vi "Collection.vi"(8 "error in (no error)":errorcluster) -> (0 "error out":errorcluster)   [LabVIEW 2017]
uses:
  Controls/First-After.ctl
  Controls/Data Save Loop States.ctl
panel:
  out "Saving Progress":u8(slide) scale=-1.0..4.0
  out "Exit?":bool
  out "Saving":bool
  out "Recording Save Path":path
  out "Recording":bool
  in  "Home Button":bool
  in  "Record Button":bool
  out "Mic 2":dynamicdata(graph)
  out "Mic 1":dynamicdata(graph)
  out "Sensor 6":dynamicdata(graph)
  out "Sensor 4":dynamicdata(graph)
  out "Sensor 3":dynamicdata(graph)
  out "Sensor 2":dynamicdata(graph)
  out "Sensor 5":dynamicdata(graph)
  out "Sensor 1":dynamicdata(graph)
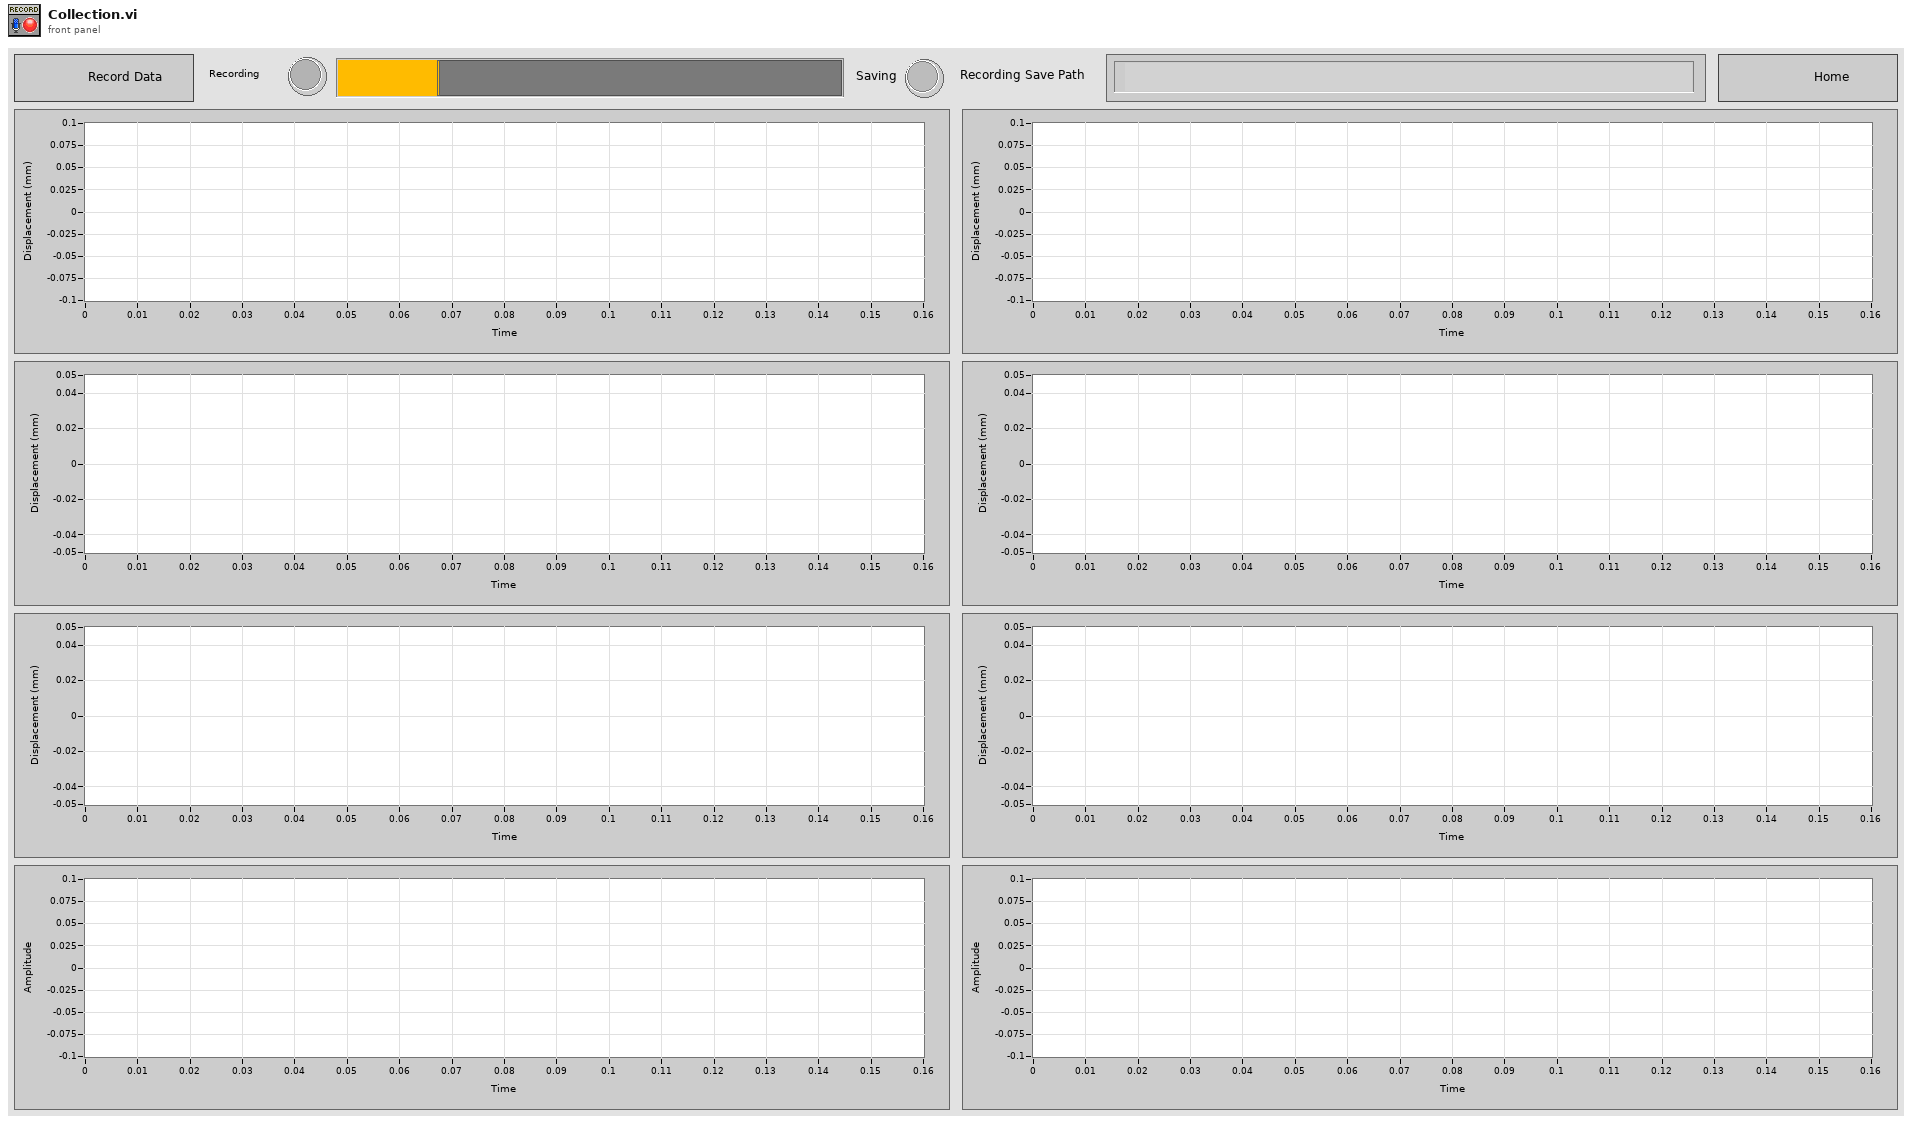
[diagram p1: front panel]
types:
  T1 = enum16{"open", "replace", "create", "open or create", "replace or create", "replace or create with confirmation"}
  T2 = typedef "Data Save Loop States.ctl" = enum16{"Waiting", "Recording", "Saving"}
  T3 = typedef "First-After.ctl" = enum16{"First", "After"}
  T4 = enum8{"Enabled", "Disabled", "Disabled and Grayed Out"}
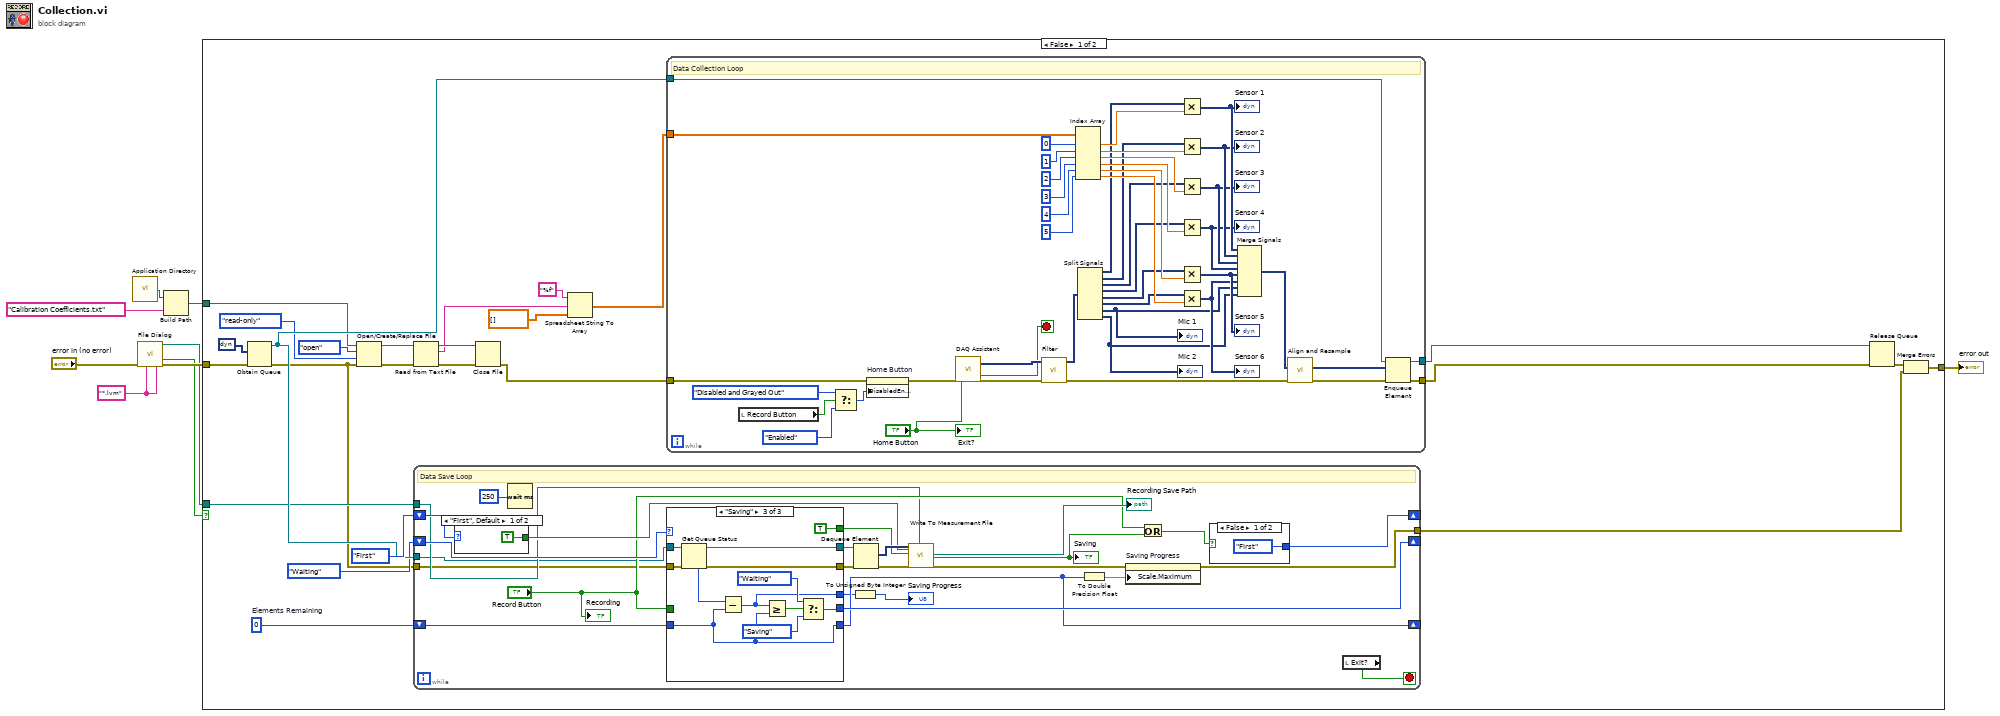
[diagram p0: block diagram]
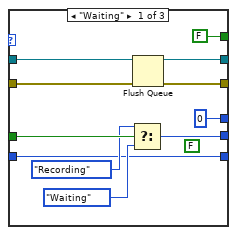
[diagram p2: hidden frame]
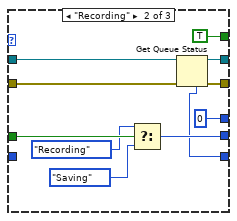
[diagram p3: hidden frame]
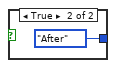
[diagram p4: hidden frame]
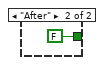
[diagram p5: hidden frame]
diagram:
  w9 = "*.lvm" ("pattern label")
  n1 = call <vilib>:"Application Directory.vi"() -> ("Application Directory"=w3:path)
  n2 = call "File Dialog"("error in"="error in (no error)", "pattern (all files)"=w9, "pattern label"=w9) -> ("selected path"=w5:path, "cancelled"=w4:bool, "error out"=w7:errorcluster)  [unwired: 9 in, 1 out]
  n3 = Build Path(base path=w3, name or relative path="Calibration Coefficients.txt") -> (appended path=w1:path)
  n4 = case shown="False" w4 {
    tunnel: w7 -> [w31 w144]
    tunnel: [w25 w144] -> w6
    tunnel: w5 -> [w24 _]
    tunnel: w1 -> [w22 _]
    frame False {
      w23 = 0  # Elements Remaining
      n5 = Obtain Queue(element data type=dynamicdata [] ("Filtered Signal"), error in (no error)=w31) -> (queue out=w32:refnum<queue>, error out=w21:errorcluster)  [unwired: 3 in, 1 out]
      n6 = Open/Create/Replace File(file path (use dialog)=w22, error in=w21, operation (0:open)=T1."open", access (0:read/write)=enum16{"read/write", "read-only", "write-only"}."read-only") -> (refnum out=w19:refnum<file>, error out=w20:errorcluster)  [unwired: 2 in, 1 out]
      n7 = Read from Text File(file (use dialog)=w19, error in=w20) -> (refnum out=w17:refnum<file>, text=w13:string, error out=w18:errorcluster)  [unwired: 2 in, 1 out]
      n8 = while {
        shift-right: [w57] -> _
        shift-left: First-After."First" -> [w59]
        tunnel: w32 -> [w35]
        tunnel: w21 -> [w36]
        shift-right: [w55] -> _
        shift-left: Data_Save_Loop_States."Waiting" -> [w56]
        tunnel: [w41] -> w26
        tunnel: w24 -> [w46]
        shift-right: [w43] -> _
        shift-left: w23 -> [w45]
        stop <- w37 stop-if-true
        # "Data Save Loop"
        n9 = case shown="\"First\", Default" w59 {
          tunnel: [TRUE FALSE] -> w53
          frame "First", Default {
          }
          frame "After" {
          }
        }
        n10 = Wait (ms)(milliseconds to wait=u32 250) -> ()  [unwired: 1 out]
        n11 = case shown="\"Saving\"" w56 {
          tunnel: "Record Button" -> [w71 w80 _]
          tunnel: [w68 w81 w91] -> w55
          tunnel: w35 -> [w63 w74 w88]
          tunnel: w36 -> [w61 w77 w87]
          tunnel: [w62 w73 w93] -> w52
          tunnel: [w64 w76 w94] -> w51
          tunnel: [FALSE TRUE TRUE] -> w50
          tunnel: [w66 w72 w83] -> w43
          tunnel: w45 -> [w66 _ w83]
          tunnel: [0 0 w84] -> w39
          frame "Waiting" {
            (unwired) FALSE ("timed out?")
            n12 = Select(t=Data_Save_Loop_States."Recording", s=w71, f=Data_Save_Loop_States."Waiting") -> (s? t:f=w68:T2)
            n13 = Flush Queue(queue=w63, error in (no error)=w61) -> (queue out=w62:refnum<queue>, error out=w64:errorcluster)  [unwired: 1 out]
          }
          frame "Recording" {
            n14 = Select(t=Data_Save_Loop_States."Recording", s=w80, f=Data_Save_Loop_States."Saving") -> (s? t:f=w81:T2)
            n15 = Get Queue Status(queue=w74, error in (no error)=w77) -> (queue out=w73:refnum<queue>, error out=w76:errorcluster, # elements in queue=w72:i32)  [unwired: 1 in, 5 out]
          }
          frame "Saving" {
            n16 = Get Queue Status(queue=w88, error in (no error)=w87) -> (queue out=w93:refnum<queue>, error out=w94:errorcluster, # elements in queue=w86:i32)  [unwired: 1 in, 5 out]
            n17 = Subtract(x=w86, y=w83) -> (x-y=w84:i32)
            n18 = Greater Or Equal?(x=w84, y=w83) -> (x >= y?=w85:bool)
            n19 = Select(t=Data_Save_Loop_States."Waiting", s=w85, f=Data_Save_Loop_States."Saving") -> (s? t:f=w91:T2)
          }
        }
        n20 = To Unsigned Byte Integer(number=w39) -> (unsigned 8bit integer=→"Saving Progress":u8)
        n21 = Dequeue Element(queue=w52, error in (no error)=w51) -> (element=w54:dynamicdata, error out=w58:errorcluster)  [unwired: 1 in, 2 out]
        n22 = call "Write To Measurement File"("Signals"=w54, "Reset"=w53, "Enable"=w50, "error in (no error)"=w58, "Filename"=w46) -> ("Filename Out"=→"Recording Save Path":path, "Saving Data"=w49:bool, "error out"=w42:errorcluster)  [unwired: 12 in]
        "Saving" <- w49
        n23 = To Double Precision Float(number=w43) -> (double precision float=w44:dbl)
        n24 = property on="Saving Progress" class="Slide (strict)"(error in=w42, "Scale.Maximum"=w44) -> (error out=w41:errorcluster)  [unwired: 1 in, 1 out]
        n25 = Or(x="Record Button", y=w49) -> (x .or. y?=w48:bool)
        n26 = case shown="False" w48 {
          tunnel: [First-After."First" First-After."After"] -> w57
          frame False {
          }
          frame True {
          }
        }
        n27 = local read "Exit?"() -> (w37:bool)
        "Recording" <- "Record Button"
      }
      n28 = Close File(refnum=w17, error in=w18) -> (error out=w16:errorcluster)  [unwired: 1 out]
      n29 = Spreadsheet String To Array(format string="%f", spreadsheet string=w13, array type (2D Dbl)=dbl[] []) -> (array=w12:dbl[])  [unwired: 1 in]
      n30 = while {
        tunnel: w16 -> [w135]
        tunnel: w32 -> [w134]
        tunnel: [w128] -> w29
        tunnel: [w127] -> w28
        tunnel: w12 -> [w126]
        stop <- w141 stop-if-true
        # "Data Collection Loop"
        n31 = local read "Record Button"() -> (w130:bool)
        n32 = Select(t=T4."Disabled and Grayed Out" ("Disabled"), s=w130, f=T4."Enabled" ("Disabled")) -> (s? t:f=w139:T4)
        n33 = property on="Home Button" class="Bool"(error in=w135, "DisabledEnum"=w139) -> (error out=w136:errorcluster)  [unwired: 1 in, 1 out]
        n34 = call "DAQ Assistant"("error in"=w136, "stop (F)"="Home Button") -> ("data"=w143:dynamicdata, "stopped"=w141:bool, "error out"=w140:errorcluster)  [unwired: 14 in, 1 out]
        n35 = call "Filter"("error in (no error)"=w140, "Signal"=w143) -> ("error out"=w133:errorcluster, "Filtered Signal"=w129:dynamicdata)  [unwired: 8 in]
        n36 = Index Array(array=w126, index #1=0 ("index"), index #2=1 ("index"), index #3=2 ("index"), index #4=3 ("index"), index #5=4 ("index"), index #6=5 ("index")) -> (element #1=w119:dbl, element #2=w118:dbl, element #3=w117:dbl, element #4=w116:dbl, element #5=w115:dbl, element #6=w114:dbl)
        n37 = Split Signals(w129) -> (w113:dynamicdata, w112:dynamicdata, w111:dynamicdata, w110:dynamicdata, w109:dynamicdata, w108:dynamicdata, w101:dynamicdata, w100:dynamicdata)  [unwired: 8 in]
        "Mic 1" <- w101
        "Mic 2" <- w100
        n38 = Multiply(x=w113, y=w119) -> (x*y=w107:dynamicdata)
        "Sensor 1" <- w107
        n39 = Multiply(x=w112, y=w118) -> (x*y=w106:dynamicdata)
        "Sensor 2" <- w106
        n40 = Multiply(x=w111, y=w117) -> (x*y=w105:dynamicdata)
        "Sensor 3" <- w105
        n41 = Multiply(x=w110, y=w116) -> (x*y=w104:dynamicdata)
        "Sensor 4" <- w104
        n42 = Multiply(x=w109, y=w115) -> (x*y=w103:dynamicdata)
        "Sensor 5" <- w103
        n43 = Multiply(x=w108, y=w114) -> (x*y=w102:dynamicdata)
        "Sensor 6" <- w102
        n44 = Merge Signals(w107, w106, w105, w104, w103, w102, w101, w100) -> (w99:dynamicdata)
        n45 = call "Align and Resample"("error in (no error)"=w133, "Signals"=w99) -> ("error out"=w132:errorcluster, "Resampled Signals"=w131:dynamicdata)  [unwired: 7 in, 1 out]
        n46 = Enqueue Element(queue=w134, element=w131, error in (no error)=w132) -> (queue out=w127:refnum<queue>, error out=w128:errorcluster)  [unwired: 1 in, 1 out]
        "Exit?" <- "Home Button"
      }
      n47 = Release Queue(queue=w28, error in (no error)=w29) -> (error out=w27:errorcluster)  [unwired: 1 in, 2 out]
      n48 = Merge Errors(w27, w26) -> (w25:errorcluster)
    }
    frame True {
    }
  }
  "error out" <- w6
